vi "Build Command.vi"(8 "error in (no error)":errorcluster, 11 "WriteCommand in":refnum<class "WriteCommand.lvclass">) -> (0 "error out":errorcluster, 2 "Command":string, 3 "WriteCommand out":refnum<class "WriteCommand.lvclass">)   [LabVIEW 2023, in "HAF.lvlib" / "WriteCommand.lvclass"]
doc: "Builds a command string up for execution on the Instrument by the Driver.  The command consists of a Base command plus any parameters that should be applied."
uses:
  WriteCommand.lvclass
  WriteCommand.lvclass/WriteCommand.ctl
  Parameter/Parameter.lvclass
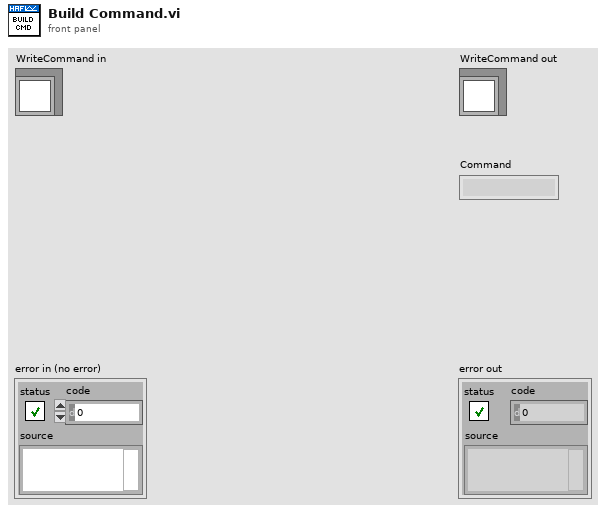
[diagram p1: front panel]
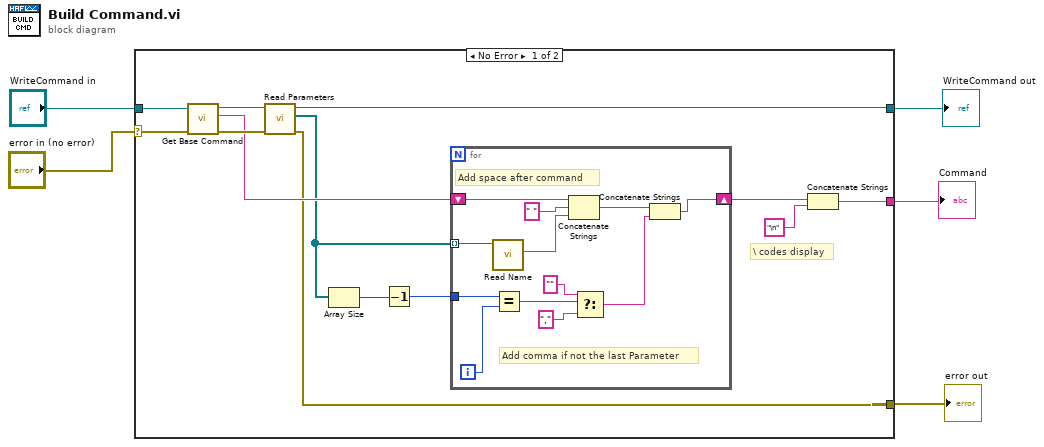
[diagram p0: block diagram]
diagram:
  n1 = case shown="No Error" "error in (no error)" {
    selector: "error in (no error)" -> [w17 w32]
    tunnel: [w6 w32] -> w4
    tunnel: [w7 w31] -> w2
    tunnel: "WriteCommand in" -> [w18 w31]
    tunnel: [w8 _] -> w1
    frame No Error {
      # "\\ codes display"
      n2 = call-dynamic "Get Base Command.vi"("error in (no error)"=w17, "WriteCommand in"=w18) -> ("error out"=w15:errorcluster, "Base Command"=w14:string, "WriteCommand out"=w16:refnum<class "WriteCommand.lvclass">)  [unwired: 7 in]
      n3 = call-dynamic "Read Parameters.vi"("error in (no error)"=w15, "WriteCommand in"=w16) -> ("error out"=w6:errorcluster, "Parameters"=w11:refnum<class "Parameter.lvclass">[], "WriteCommand out"=w7:refnum<class "WriteCommand.lvclass">)  [unwired: 7 in]
      n4 = Array Size(array=w11) -> (size(s)=w13:i32)
      n5 = Decrement(x=w13) -> (x-1=w12:i32)
      n6 = for {
        tunnel: w12 -> [w26]
        tunnel: w11 -> [w30] mode=indexing
        shift-right: [w19] -> w10
        shift-left: w14 -> [w29]
        i -> [w25]
        # "Add space after command"
        # "Add comma if not the last Parameter"
        n7 = call-dynamic "Read Name.vi"("Parameter in"=w30) -> ("Name"=w27:string)  [unwired: 8 in, 2 out]
        n8 = Equal?(x=w26, y=w25) -> (x = y?=w24:bool)
        n9 = Concatenate Strings(w29, " " ("string"), w27) -> (w21:string)
        n10 = Select(t="", s=w24, f=",") -> (s? t:f=w20:string)
        n11 = Concatenate Strings(w21, w20) -> (w19:string)
      }
      n12 = Concatenate Strings(w10, "\n" ("string")) -> (w8:string)
    }
    frame Error {
    }
  }
  "error out" <- w4
  "WriteCommand out" <- w2
  "Command" <- w1
